vi "1 CNT.vi"(6 "m-nm l":dbl, 9 "Length of CNTs":dbl, 10 "m-nm r":dbl, 11 "Radius of CNTs":dbl) -> (0 "Length of CNTs":dbl, 1 "Surface Area of 1 CNT":dbl, 2 "CNT Base Area":dbl, 3 "CNT Radius":dbl)   [LabVIEW 2020]
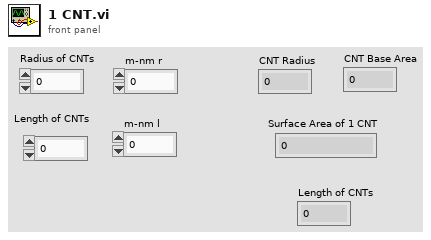
[diagram p1: front panel]
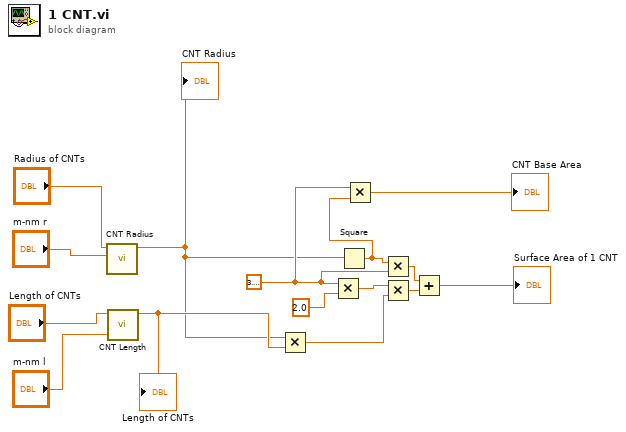
[diagram p0: block diagram]
diagram:
  w15 = 3.141592653589793
  n1 = call "CNT Radius.vi"("m-nm r"="m-nm r", "Radius of CNTs"="Radius of CNTs") -> ("Numeric"=w10:dbl)  [unwired: 9 in]
  "CNT Radius" <- w10
  n2 = call "CNT Length.vi"("m-nm l"="m-nm l", "Length of CNTs"="Length of CNTs") -> ("Numeric"=w11:dbl)  [unwired: 9 in]
  "Length of CNTs" <- w11
  n3 = Multiply(x=w10, y=w11) -> (x*y=w7:dbl)
  n4 = Multiply(x=w15, y=2.0) -> (x*y=w6:dbl)
  n5 = Square(x=w10) -> (x^2=w14:dbl)
  n6 = Multiply(x=w15, y=w14) -> (x*y=→"CNT Base Area":dbl)
  n7 = Multiply(x=w14, y=w15) -> (x*y=w9:dbl)
  n8 = Multiply(x=w6, y=w7) -> (x*y=w8:dbl)
  n9 = Add(x=w9, y=w8) -> (x+y=→"Surface Area of 1 CNT":dbl)
